vi "log.vi"(7 "severity":T1, 8 "error in (no error)":errorcluster, 10 "message":string) -> (0 "error out":errorcluster)   [LabVIEW 2021, in "system.logging.lvclass"]
uses:
  system.logging.lvclass
  severity.ctl
  log_entry.ctl
  system.logging.lvclass/system.logging.ctl
  service_commands.ctl
  log_stream.ctl
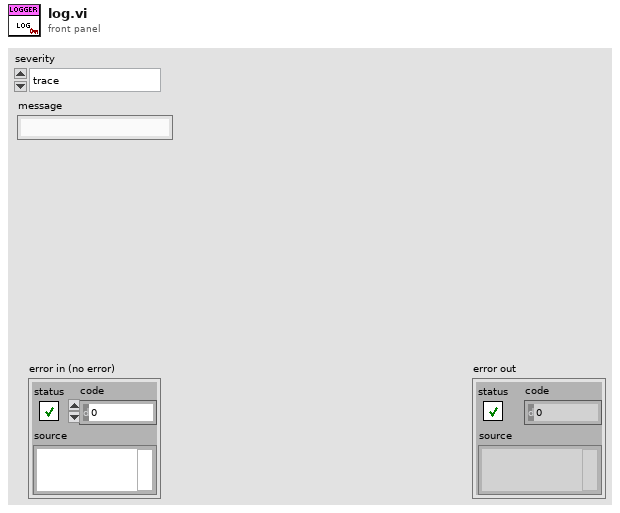
[diagram p1: front panel]
types:
  T1 = typedef "system.logging.lvclass/severity.ctl" = enum8{"trace", "debug", "info", "warning", "error"}
  T2 = typedef "system.logging.lvclass/log_stream.ctl" = cluster{"command":T3, "log_entry":T4}
  T3 = typedef "system.logging.lvclass/service_commands.ctl" = enum16{"close", "log"}
  T4 = typedef "system.logging.lvclass/log_entry.ctl" = cluster{"severity":T1, "message":string, "origin":string, "datetime":timestamp}
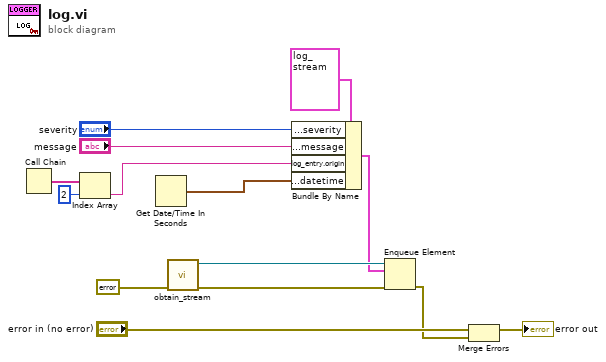
[diagram p0: block diagram]
diagram:
  n1 = Call Chain() -> (call chain=w8:string[])
  n2 = Index Array(array=w8, index=2) -> (element=w3:string)
  n3 = Get Date/Time In Seconds() -> (seconds since 1Jan1904=w2:timestamp)
  n4 = call "obtain_stream.vi"("error in (no error)"=errorcluster {"status"=FALSE, "code"=0, "source"=""}) -> ("error out"=w13:errorcluster, "log_stream"=w12:refnum<queue>)  [unwired: 9 in]
  n5 = Bundle By Name(cluster=T2 {"command"=enum."log", "log_entry"={"severity"=enum."trace", "message"="", "origin"="", "datetime"=timestamp(0 s since 1904-01-01)}} ("log_stream"), "log_entry.severity"="severity", "log_entry.message"="message", "log_entry.origin"=w3, "log_entry.datetime"=w2) -> (w1:T2)
  n6 = Enqueue Element(queue=w12, element=w1, error in (no error)=w13) -> (error out=w10:errorcluster)  [unwired: 1 in, 2 out]
  n7 = Merge Errors("error in (no error)", w10) -> (→"error out":errorcluster)
